vi "SL2_AD_DLL_Phoibos_ListVoltages.vi"(0 "dll path in":path, 2 "pHandle":u32, 3 "error in":errorcluster) -> (5 "dll path out":path, 6 "voltage_infos":T1[](array[typedef]), 7 "voltage_names":string[](array[string]), 8 "error out":errorcluster)   [LabVIEW 2015]
uses:
  DEFINITIONS/DEF_voltage_info.ctl
  DEFINITIONS/DEF_T_error_enum.ctl
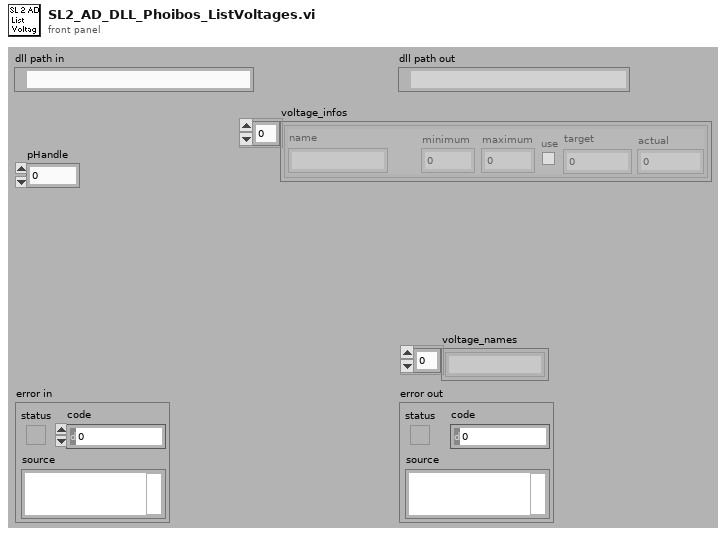
[diagram p1: front panel]
types:
  T1 = typedef "DEF_voltage_info.ctl" = cluster{"name":string, "maximum":dbl, "minimum":dbl, "actual":dbl, "use":bool, "target":dbl}
  T2 = enum16{"open", "replace", "create", "open or create", "replace or create", "replace or create with confirmation"}
  T3 = typedef "DEF_T_error_enum.ctl" = u32
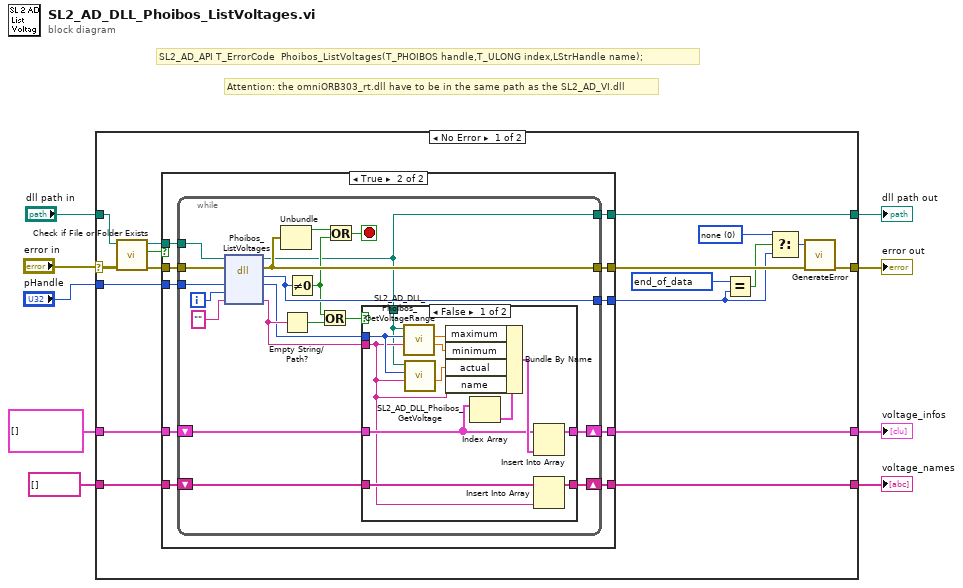
[diagram p0: block diagram]
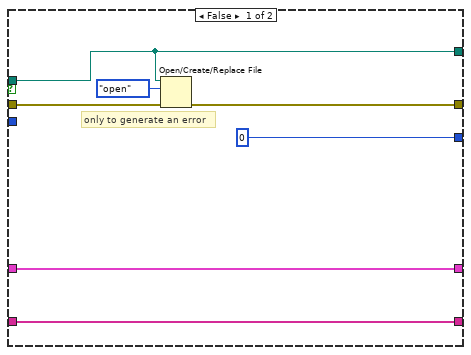
[diagram p2: hidden frame]
diagram:
  # "SL2_AD_API T_ErrorCode  Phoibos_ListVoltages(T_PHOIBOS handle,T_ULONG index,LStrHandle name);"
  # "Attention: the omniORB303_rt.dll have to be in the same path as the SL2_AD_VI.dll"
  n1 = case shown="No Error" "error in" {
    selector: "error in" -> [w25 w80]
    tunnel: [w27 w79] -> w4
    tunnel: [w18 w80] -> w9
    tunnel: [w26 w81] -> w8
    tunnel: "dll path in" -> [w24 w81]
    tunnel: "pHandle" -> [w23 _]
    tunnel: [w22 w78] -> w3
    tunnel: string[] [] ("Array") -> [w21 w79]
    tunnel: T1[] [] -> [w20 w78]
    frame No Error {
      w15 = T3 8388608 items=["none"=0, "busy"=65536, "error"=131072, "parameter"=262144, "locked"=524288, "sync"=1048576, "connection"=2097152, "internal"=4194304, "end_of_data"=8388608] ("DEF_T_error_enum")
      w16 = T3 0 items=["none"=0, "busy"=65536, "error"=131072, "parameter"=262144, "locked"=524288, "sync"=1048576, "connection"=2097152, "internal"=4194304, "end_of_data"=8388608] ("DEF_T_error_enum")
      n2 = call <vilib>:"Check if File or Folder Exists.vi"("error in (no error)"=w25, "path"=w24) -> ("error out"=w10:errorcluster, "file or folder exists?"=w12:bool, "dup path"=w11:path)  [unwired: 7 in]
      n3 = case shown="True" w12 {
        tunnel: [w33 w44] -> w27
        tunnel: [w31 w43] -> w19
        tunnel: [0 ("error_code") w42] -> w13
        tunnel: [w29 w41] -> w26
        tunnel: w11 -> [w29 w40]
        tunnel: w10 -> [w32 w39]
        tunnel: w21 -> [w33 w38]
        tunnel: w23 -> [_ w37]
        tunnel: [w28 w36] -> w22
        tunnel: w20 -> [w28 w35]
        frame False {
          # "only to generate an error"
          n4 = Open/Create/Replace File(file path (use dialog)=w29, error in=w32, operation (0:open)=T2."open") -> (error out=w31:errorcluster)  [unwired: 3 in, 2 out]
        }
        frame True {
          n5 = while {
            tunnel: [w55] -> w42
            tunnel: [w60] -> w43
            shift-right: [w46] -> w44
            shift-left: w38 -> [w48]
            tunnel: w40 -> [w59]
            tunnel: w39 -> [w61]
            tunnel: [w45] -> w41
            tunnel: w37 -> [w58]
            shift-right: [w47] -> w36
            shift-left: w35 -> [w50]
            i -> [w57]
            stop <- w63 stop-if-true
            n6 = dll-call lib="C:/Programme/SPECS/SpecsLab2/programming/LabView7.1/SL2_AD_VI.dll" fn="Phoibos_ListVoltages" ("ListVoltages")(path in=w59, error in=w61, "pHandle"=w58, "index"=w57, "modeName"="") -> (path out=w45:path, error out=w60:errorcluster, "errorCode"=w55:u32, "pHandle"=w51:u32, "modeName"=w52:string)  [unwired: 2 in]
            n7 = Unbundle(w60) -> ("status"=w62:bool)  [unwired: 2 out]
            n8 = Empty String/Path?(string/path=w52) -> (empty?=w53:bool)
            n9 = Not Equal To 0?(x=w55) -> (x != 0?=w54:bool)
            n10 = Or(x=w54, y=w53) -> (x .or. y?=w49:bool)
            n11 = Or(x=w62, y=w54) -> (x .or. y?=w63:bool)
            n12 = case shown="False" w49 {
              tunnel: [w75 w77] -> w46
              tunnel: w48 -> [w74 w77]
              tunnel: w50 -> [w67 w76]
              tunnel: [w73 w76] -> w47
              tunnel: w52 -> [w65 _]
              tunnel: w51 -> [w68 _]
              tunnel: w45 -> [w64 _]
              frame False {
                n13 = call "SL2_AD_DLL_Phoibos_GetVoltageRange.vi"("voltage_name"=w65, "pHandle"=w68, "dll path in"=w64) -> ("min"=w72:dbl, "max"=w70:dbl)  [unwired: 3 in, 2 out]
                n14 = call "SL2_AD_DLL_Phoibos_GetVoltage.vi"("voltage_name"=w65, "pHandle"=w68, "dll path in"=w64) -> ("value"=w71:dbl)  [unwired: 4 in, 2 out]
                n15 = Index Array(array=w67) -> (element=w66:T1)  [unwired: 1 in]
                n16 = Bundle By Name(cluster=w66, "maximum"=w70, "minimum"=w72, "actual"=w71, "name"=w65) -> (w69:T1)
                n17 = Insert Into Array(array=w67, new element=w69) -> (w73:T1[])  [unwired: 1 in]
                n18 = Insert Into Array(array=w74, new element=w65) -> (w75:string[])  [unwired: 1 in]
              }
              frame True {
              }
            }
          }
        }
      }
      n19 = Equal?(x=w15, y=w13) -> (x = y?=w14:bool)
      n20 = Select(t=w16, s=w14, f=w13) -> (s? t:f=w17:T3)
      n21 = call "GenerateError.vi"("error in"=w19, "error_code"=w17) -> ("error out"=w18:errorcluster)  [unwired: 9 in]
    }
    frame Error {
    }
  }
  "voltage_names" <- w4
  "error out" <- w9
  "dll path out" <- w8
  "voltage_infos" <- w3
